vi "Generate Images Event.vi"(8 "error in (no error)":errorcluster, 10 "OutputDirPath":path, 11 "DLP2 in":refnum<class "DLP2.lvclass">) -> (0 "error out":errorcluster, 3 "DLP2 out":refnum<class "DLP2.lvclass">)   [LabVIEW 2022 SP3, in "DLP2.lvclass"]
doc: "Developed by Kevin Thompson\nkevin@thompsonengineering.net\n\nCopyright 2018\nThompson Engineering, LLC"
uses:
  DLP2.lvclass
  DLP2.lvclass/DLP2.ctl
  Accessors/Get PublicEvents.vi
  DataTypes/Images--Cluster.ctl
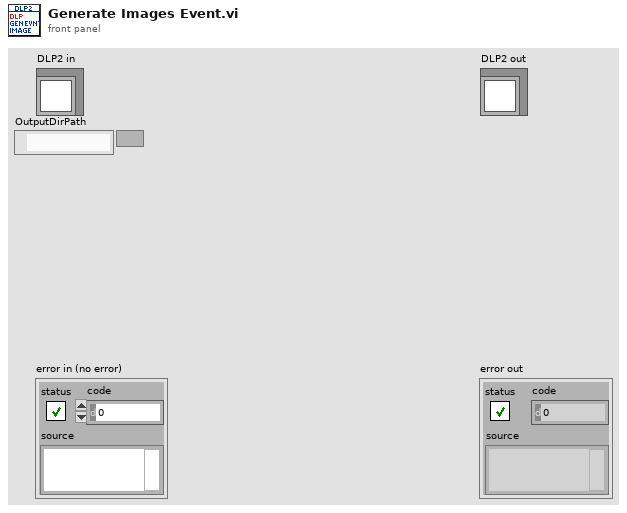
[diagram p1: front panel]
types:
  T1 = typedef "Images--Cluster.ctl" = cluster{"OutputDirPath":path}
  T2 = typedef "DLP2.lvclass/Public Events--cluster.ctl" = cluster{"Temp01.AsyncCmd Event":refnum<user-event>, "Temp01.AsyncMsg Event":refnum<user-event>, "stop process":refnum<user-event>, "API Incoming Event":refnum<user-event>, "API Executed Event":refnum<user-event>, "API Return Event":refnum<user-event>, "Images":refnum<user-event>}
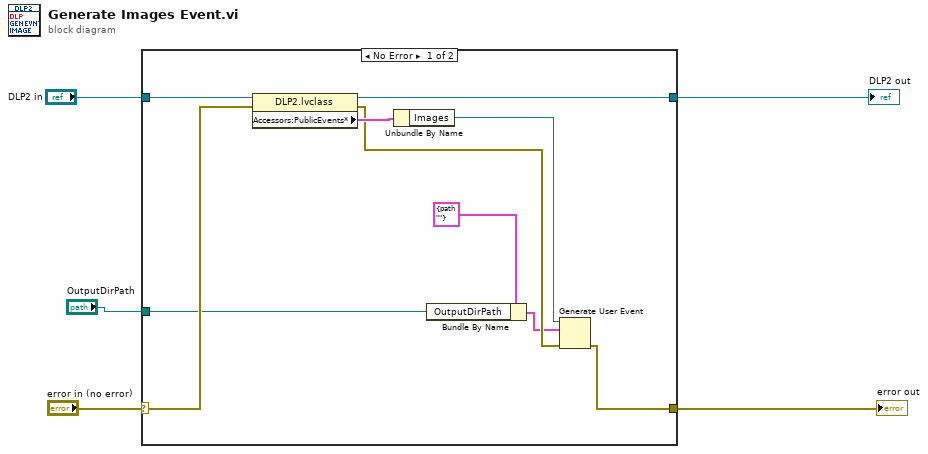
[diagram p0: block diagram]
diagram:
  n1 = case shown="No Error" "error in (no error)" {
    selector: "error in (no error)" -> [w12 w17]
    tunnel: [w10 w17] -> w4
    tunnel: [w14 w16] -> w2
    tunnel: "DLP2 in" -> [w15 w16]
    tunnel: "OutputDirPath" -> [w6 _]
    frame No Error {
      n2 = property class="DLP2.lvclass"(reference=w15, error in=w12) -> (reference out=w14:refnum<class "DLP2.lvclass">, error out=w9:errorcluster, "Accessors:PublicEvents*"=w13:T2)
      n3 = Unbundle By Name(w13) -> ("Images"=w11:refnum<user-event>)
      n4 = Bundle By Name(cluster=T1 {"OutputDirPath"=path ""} ("event data"), "OutputDirPath"=w6) -> (w7:T1)
      n5 = Generate User Event(user event=w11, event data cluster=w7, error in=w9) -> (error out=w10:errorcluster)  [unwired: 1 in, 1 out]
    }
    frame Error {
    }
  }
  "error out" <- w4
  "DLP2 out" <- w2
